vi "ZControlCam2.vi"() -> ()   [LabVIEW 2014]
uses:
  <vilib>/vision/Vision Builder AI/API.llb/IVB Interface - VBAI Version.ctl
  <vilib>/vision/Vision Builder AI/API.llb/VBAI Interface - Get Inspection Image (By Name).vi
panel:
  out "PASS/FAIL Flag":bool
  out "decimal integer string":string
  in  "Boolean":bool
  out "Defence 1 Y":dbl
  out "Defence 1 X":dbl
  out "MatchBall Y":dbl
  out "MatchBallX":dbl
  out "Kicker Y":dbl
  out "Kicker X":dbl format="%_3g"
  out "Image":T1(plugin-control)
  in  "stop":bool
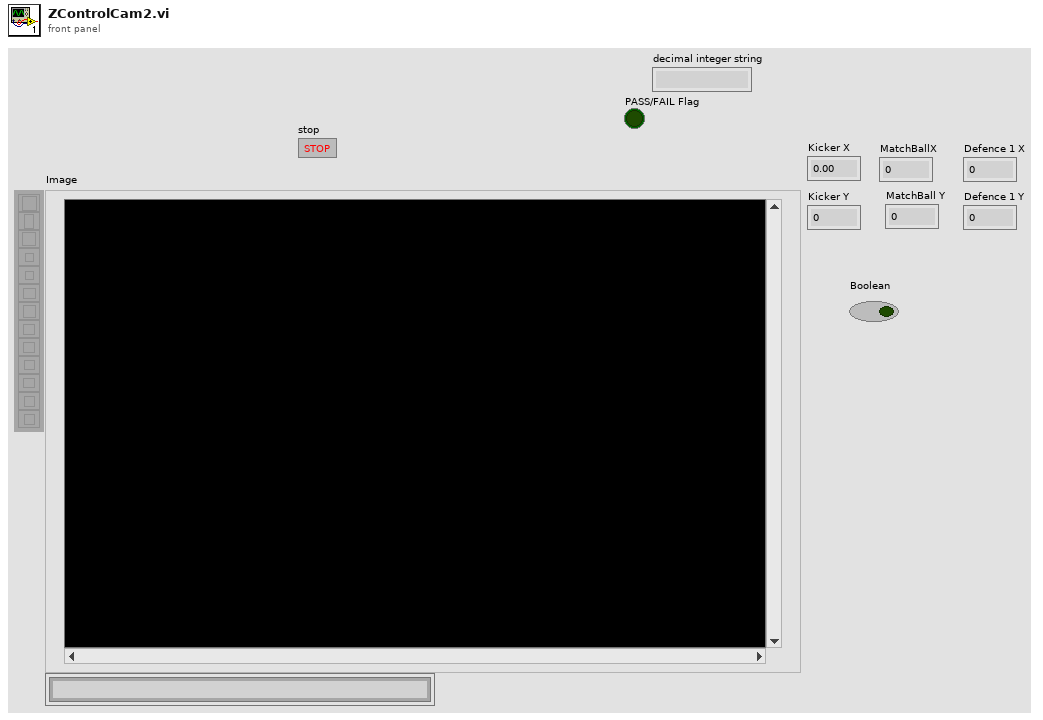
[diagram p1: front panel]
types:
  T1 = typedef "IMAQ Image.ctl" = refnum<image>
  T2 = typedef "Image Type" = u32
  T3 = typedef "IVB Interface - VBAI Version.ctl" = u16
  T4 = typedef "VBAIInterface.ctl" = refnum<k21>
  T5 = cluster{"PASS/FAIL Flag":bool, "Numeric Measurement":dbl, "String Measurement":string, "Report Text":string}[]
  T6 = cluster{"PASS/FAIL Flag":bool, "Numeric Measurement":dbl, "String Measurement":string, "Report Text":string}
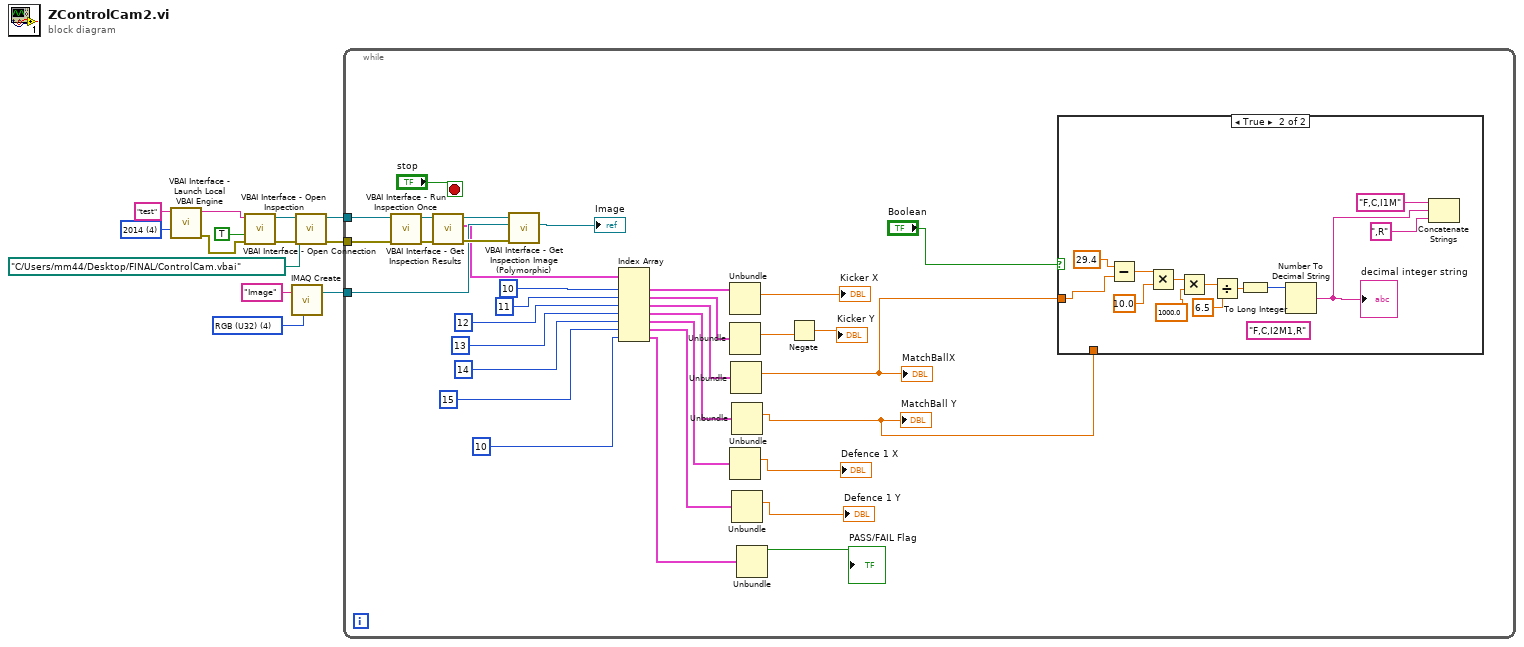
[diagram p0: block diagram]
diagram:
  w2 = T2 4 items=["Grayscale (U8)", "Grayscale (I16)", "Grayscale (SGL)", "Complex (CSG)", "RGB (U32)", "HSL (U32)", "RGB (U64)", "Grayscale (U16)"] ("Image Type")
  w10 = T3 4 items=["2010", "2011", "2012", "2013", "2014"] ("Engine Version")
  n1 = call <vilib>:"VBAI Interface - Launch Local VBAI Engine.vi"("Engine Version"=w10, "Local VBAI Engine Name"="test") -> ("error out"=w1:errorcluster, "Session Name Out"=w11:string)  [unwired: 8 in]
  n2 = call <vilib>:"VBAI Interface - Open Connection.vi"("error in"=w1, "Force Connection (False)"=TRUE, "Session In"=w11) -> ("error out"=w9:errorcluster, "Session Out"=w8:T4)  [unwired: 7 in]
  n3 = call "IMAQ Create"("Image Name"="Image", "Image Type"=w2) -> ("New Image"=w4:T1)  [unwired: 3 in, 1 out]
  n4 = call <vilib>:"VBAI Interface - Open Inspection.vi"("error in"=w9, "Path"=path "C:/Users/mm44/Desktop/FINAL/ControlCam.vbai", "Session In"=w8) -> ("error out"=w5:errorcluster, "Session Out"=w6:T4)  [unwired: 7 in]
  n5 = while {
    tunnel: w6 -> [w44]
    tunnel: w5 -> [w43]
    tunnel: w4 -> [w39]
    stop <- "stop" stop-if-true
    n6 = call <vilib>:"VBAI Interface - Run Inspection Once.vi"("error in"=w43, "Session In"=w44) -> ("error out"=w46:errorcluster, "Session Out"=w45:T4)  [unwired: 8 in]
    n7 = call <vilib>:"VBAI Interface - Get Inspection Results.vi"("error in"=w46, "Session In"=w45) -> ("error out"=w40:errorcluster, "Step Results"=w37:T5, "Session Out"=w41:T4)  [unwired: 3 in, 4 out]
    n8 = call-poly <vilib>:"VBAI Interface - Get Inspection Image (Polymorphic).vi"("error in"=w40, "Image Dest"=w39, "Session In"=w41) -> ("Image Dst Out"=→"Image":T1)  [unwired: 5 in, 3 out]
    n9 = Index Array(array=w37, index #1=10 ("index"), index #2=11 ("index"), index #3=12 ("index"), index #4=13 ("index"), index #5=14 ("index"), index #6=15 ("index"), index #7=10 ("index")) -> (element #1=w36:T6, element #2=w33:T6, element #3=w25:T6, element #4=w24:T6, element #5=w23:T6, element #6=w22:T6, element #7=w16:T6)
    n10 = Unbundle(w36) -> ("Numeric Measurement"=→"Kicker X":dbl)  [unwired: 3 out]
    n11 = Unbundle(w33) -> ("Numeric Measurement"=w32:dbl)  [unwired: 3 out]
    n12 = Unbundle(w23) -> ("Numeric Measurement"=→"Defence 1 X":dbl)  [unwired: 3 out]
    n13 = Unbundle(w25) -> ("Numeric Measurement"=w18:dbl)  [unwired: 3 out]
    "MatchBallX" <- w18
    n14 = Unbundle(w24) -> ("Numeric Measurement"=w17:dbl)  [unwired: 3 out]
    "MatchBall Y" <- w17
    n15 = Unbundle(w22) -> ("Numeric Measurement"=→"Defence 1 Y":dbl)  [unwired: 3 out]
    n16 = Unbundle(w16) -> ("PASS/FAIL Flag"=→"PASS/FAIL Flag":bool)  [unwired: 3 out]
    n17 = Negate(x=w32) -> (-x=→"Kicker Y":dbl)
    n18 = case shown="True" "Boolean" {
      tunnel: w18 -> [_ w56]
      tunnel: w17 -> [_ _]
      frame False {
      }
      frame True {
        (unwired) "F,C,I2M1,R" ("string")
        n19 = Subtract(x=29.4, y=w56) -> (x-y=w55:dbl)
        n20 = Multiply(x=w55, y=10.0) -> (x*y=w53:dbl)
        n21 = Multiply(x=w53, y=1000.0) -> (x*y=w51:dbl)
        n22 = Divide(x=w51, y=6.5) -> (x/y=w49:dbl)
        n23 = To Long Integer(number=w49) -> (32bit integer=w48:i32)
        n24 = Number To Decimal String(number=w48) -> (decimal integer string=w47:string)  [unwired: 1 in]
        "decimal integer string" <- w47
        n25 = Concatenate Strings("F,C,I1M" ("string"), w47, ",R" ("string")) -> ()  [unwired: 1 out]
      }
    }
  }
